vi "Create Table.vi"(8 "error in (no error)":errorcluster, 11 "Access in":refnum<class "Access.lvclass">) -> (0 "error out":errorcluster, 3 "Access out":refnum<class "Access.lvclass">)   [LabVIEW 2016, in "Database.lvlib" / "Access.lvclass"]
uses:
  Access.lvclass
  <vilib>/addons/database/NI_Database_API.lvlib
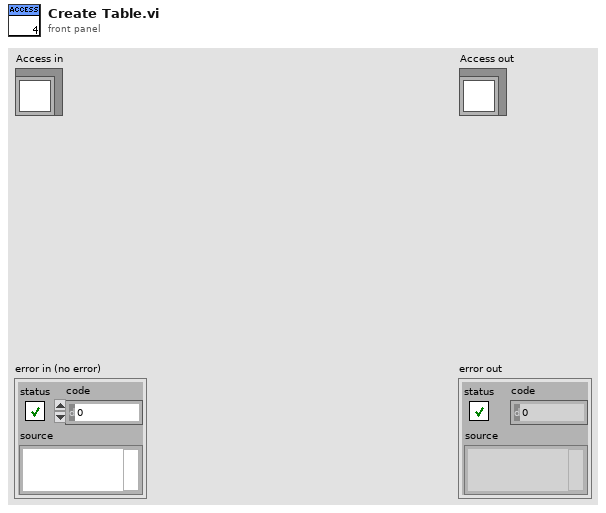
[diagram p1: front panel]
types:
  T1 = typedef "Database.lvlib/DB.lvclass/Column_info.ctl" = cluster{"Authentication":T2[], "Instr_Configuration":T2[], "Recipe":T2[], "Test_data":T2[]}
  T2 = typedef "NI_Database_API.lvlib/DB Tools Column Info.ctl" = cluster{"column name":string, "data type":T3, "size":i32, "allow null?":bool}
  T3 = typedef "NI_Database_API.lvlib/DB Tools DataTypes.ctl" = enum16{"String", "Long (I32)", "Single (SGL)", "Double (DBL)", "Date/Time", "Binary"}
  T4 = typedef "Database.lvlib/DB.lvclass/Table_info.ctl" = cluster{"Authentication":string, "Instr_Configuration":string, "Recipe":string, "Test_data":string}
  T5 = typedef "NI_Database_API.lvlib/Conn ObjectReference.ctl" = refnum<k1>
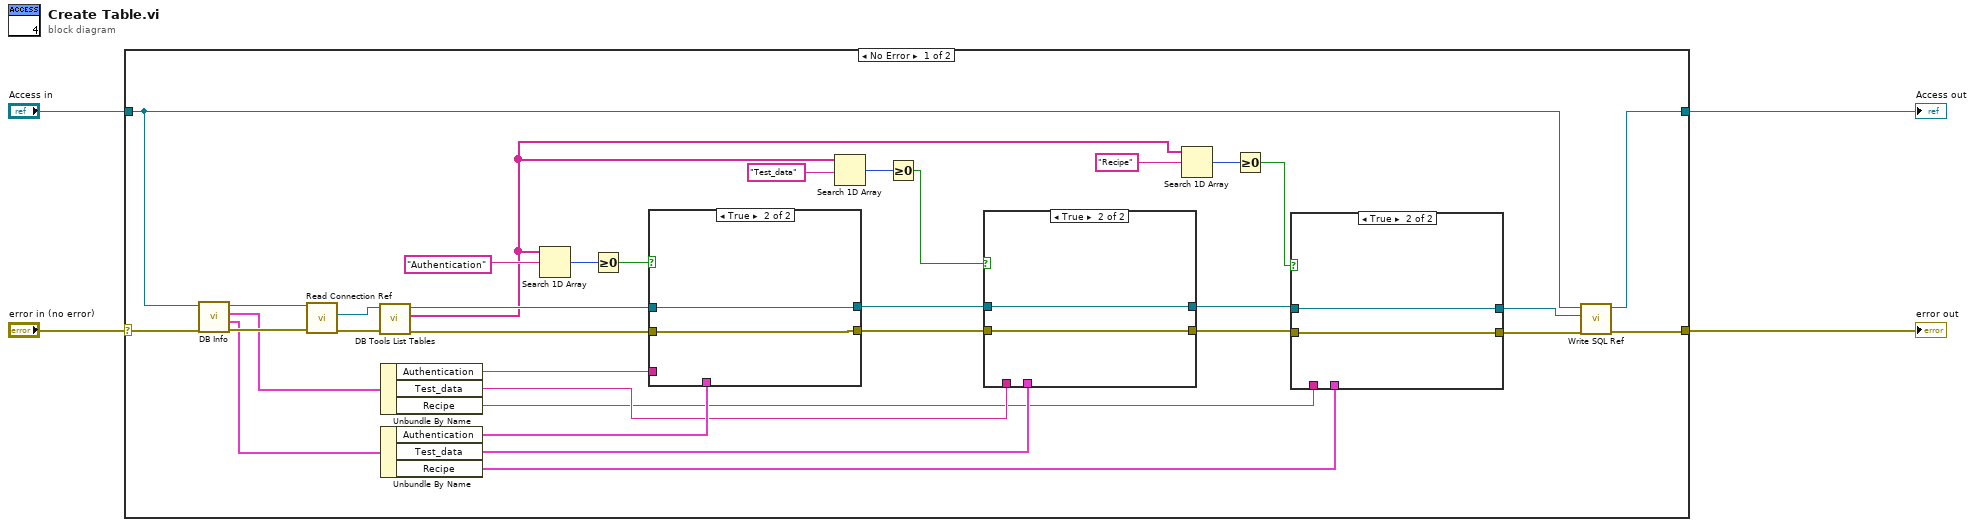
[diagram p0: block diagram]
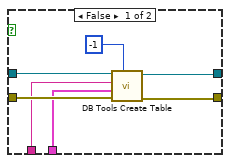
[diagram p2: hidden frame]
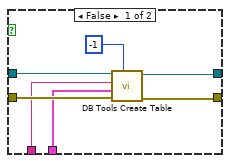
[diagram p3: hidden frame]
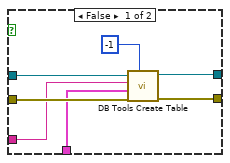
[diagram p4: hidden frame]
diagram:
  n1 = case shown="No Error" "error in (no error)" {
    selector: "error in (no error)" -> [w38 w66]
    tunnel: "Access in" -> [w30 w67]
    tunnel: [w31 w66] -> w2
    tunnel: [w29 w67] -> w1
    frame No Error {
      n2 = call-dynamic "DB Info.vi"("error in (no error)"=w38, "Access in"=w30) -> ("error out"=w36:errorcluster, "Column_info"=w34:T1, "Table_info"=w35:T4, "Access out"=w37:refnum<class "Access.lvclass">)  [unwired: 6 in]
      n3 = call-dynamic "Read Connection Ref.vi"("error in (no error)"=w36, "Access in"=w37) -> ("error out"=w32:errorcluster, "connection reference"=w33:T5)  [unwired: 7 in, 1 out]
      n4 = call <vilib>:"DB Tools List Tables.vi"("error in (no error)"=w32, "connection reference"=w33) -> ("error out"=w28:errorcluster, "tables"=w14:string[], "connection reference out"=w24:T5)  [unwired: 3 in]
      n5 = Unbundle By Name(w35) -> ("Authentication"=w23:string, "Test_data"=w16:string, "Recipe"=w8:string)
      n6 = Unbundle By Name(w34) -> ("Authentication"=w22:T2[], "Test_data"=w15:T2[], "Recipe"=w7:T2[])
      n7 = Search 1D Array(1D array=w14, element="Authentication") -> (index of element=w26:i32)  [unwired: 1 in]
      n8 = Greater Or Equal To 0?(x=w26) -> (x >= 0?=w25:bool)
      n9 = case shown="True" w25 {
        tunnel: w28 -> [w62 w64]
        tunnel: w24 -> [w61 w65]
        tunnel: w23 -> [w60 _]
        tunnel: w22 -> [w59 _]
        tunnel: [w58 w64] -> w18
        tunnel: [w57 w65] -> w17
        frame False {
          n10 = call <vilib>:"DB Tools Create Table.vi"("primary key (-1)"=-1, "error in (no error)"=w62, "column information"=w59, "table"=w60, "connection reference"=w61) -> ("error out"=w58:errorcluster, "connection reference out"=w57:T5)  [unwired: 3 in]
        }
        frame True {
        }
      }
      n11 = Search 1D Array(1D array=w14, element="Test_data") -> (index of element=w21:i32)  [unwired: 1 in]
      n12 = Greater Or Equal To 0?(x=w21) -> (x >= 0?=w19:bool)
      n13 = case shown="True" w19 {
        tunnel: w18 -> [w53 w55]
        tunnel: w17 -> [w52 w56]
        tunnel: w16 -> [w51 _]
        tunnel: w15 -> [w50 _]
        tunnel: [w49 w56] -> w10
        tunnel: [w48 w55] -> w9
        frame False {
          n14 = call <vilib>:"DB Tools Create Table.vi"("primary key (-1)"=-1, "error in (no error)"=w53, "column information"=w50, "table"=w51, "connection reference"=w52) -> ("error out"=w48:errorcluster, "connection reference out"=w49:T5)  [unwired: 3 in]
        }
        frame True {
        }
      }
      n15 = Search 1D Array(1D array=w14, element="Recipe") -> (index of element=w12:i32)  [unwired: 1 in]
      n16 = Greater Or Equal To 0?(x=w12) -> (x >= 0?=w11:bool)
      n17 = case shown="True" w11 {
        tunnel: w9 -> [w44 w46]
        tunnel: w10 -> [w43 w47]
        tunnel: w8 -> [w42 _]
        tunnel: w7 -> [w41 _]
        tunnel: [w40 w47] -> w5
        tunnel: [w39 w46] -> w6
        frame False {
          n18 = call <vilib>:"DB Tools Create Table.vi"("primary key (-1)"=-1, "error in (no error)"=w44, "column information"=w41, "table"=w42, "connection reference"=w43) -> ("error out"=w39:errorcluster, "connection reference out"=w40:T5)  [unwired: 3 in]
        }
        frame True {
        }
      }
      n19 = call-dynamic "Write SQL Ref.vi"("error in (no error)"=w6, "connection reference"=w5, "Access in"=w30) -> ("error out"=w31:errorcluster, "Access out"=w29:refnum<class "Access.lvclass">)  [unwired: 7 in]
    }
    frame Error {
    }
  }
  "error out" <- w2
  "Access out" <- w1
